vi "Logger Write.vi"(6 "Extra":string, 8 "error in (no error)":errorcluster, 9 "Command":string, 10 "State":string, 11 "Logger in":refnum<class "Logger.lvclass">) -> (0 "error out":errorcluster)   [LabVIEW 2019, in "TS Framework.lvlib" / "Logger.lvclass"]
uses:
  Logger.lvclass
  Logger.lvclass/Logger.ctl
  <vilib>/Utility/error.llb/DialogType.ctl
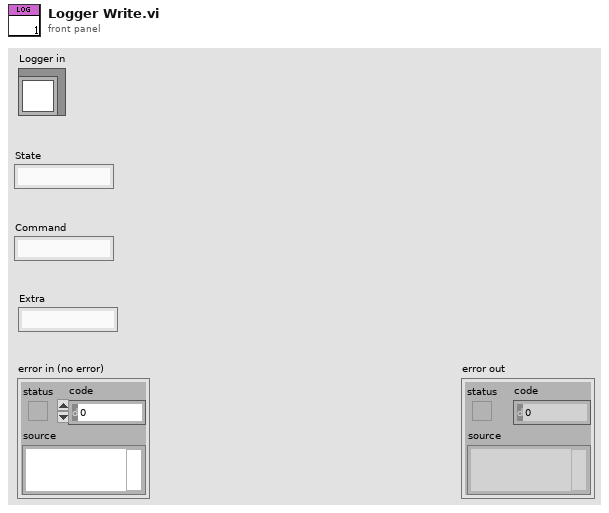
[diagram p1: front panel]
types:
  T1 = typedef "DialogType.ctl" = u16
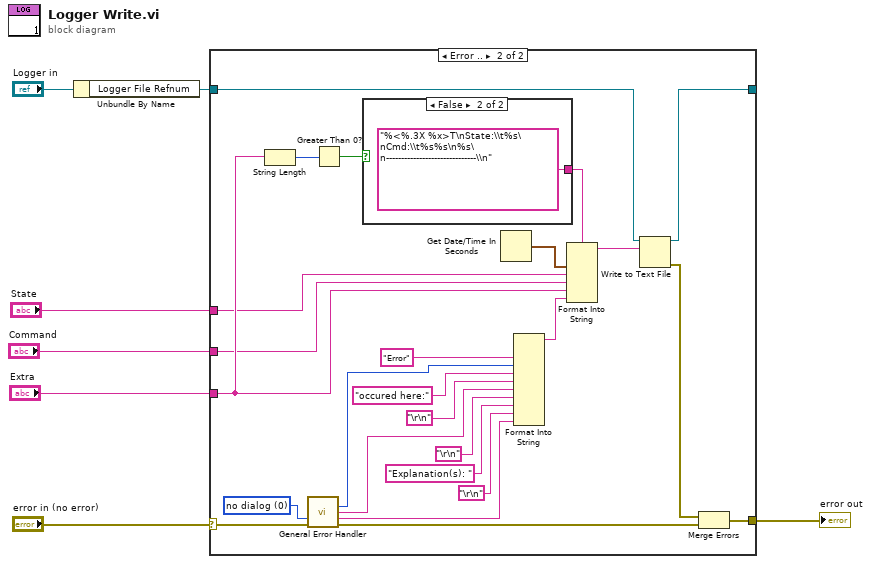
[diagram p0: block diagram]
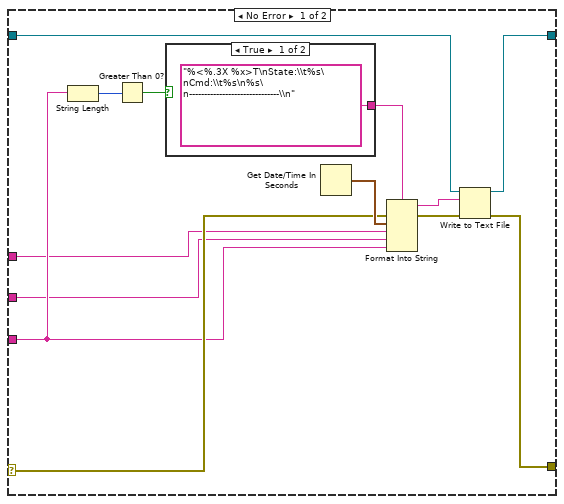
[diagram p2: hidden frame]
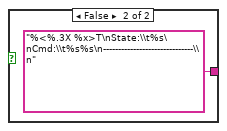
[diagram p3: hidden frame]
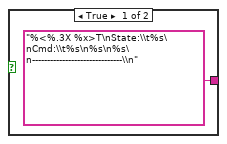
[diagram p4: hidden frame]
diagram:
  n1 = Unbundle By Name("Logger in") -> ("Logger File Refnum"=w5:refnum<file>)
  n2 = case shown="Error .." "error in (no error)" {
    selector: "error in (no error)" -> [w13 w36]
    tunnel: w5 -> [w17 w38]
    tunnel: [w16 w37] -> _
    tunnel: [w15 w33] -> w2
    tunnel: "Extra" -> [w10 w28]
    tunnel: "State" -> [w9 w25]
    tunnel: "Command" -> [w8 w26]
    frame No Error {
      n3 = String Length(string=w10) -> (length=w11:i32)
      n4 = Greater Than 0?(x=w11) -> (x > 0?=w12:bool)
      n5 = case shown="True" w12 {
        tunnel: ["%<%.3X %x>T\nState:\\t%s\nCmd:\\t%s\n%s\n------------------------------\\n" ("format string") "%<%.3X %x>T\nState:\\t%s\nCmd:\\t%s%s\n------------------------------\\n" ("format string")] -> w18
        frame True {
        }
        frame False {
        }
      }
      n6 = Get Date/Time In Seconds() -> (seconds since 1Jan1904=w19:timestamp)
      n7 = Format Into String(format string=w18, error in=w13, w19, w9, w8, w10) -> (resulting string=w20:string, error out=w14:errorcluster)  [unwired: 1 in]
      n8 = Write to Text File(file (use dialog)=w17, text=w20, error in=w14) -> (refnum out=w16:refnum<file>, error out=w15:errorcluster)  [unwired: 1 in, 1 out]
    }
    frame Error {
      w24 = T1 0 items=["no dialog", "OK message", "continue or stop message", "OK message + warnings", "continue/stop + warnings"] ("type of dialog (OK msg:1)")
      n9 = String Length(string=w28) -> (length=w29:i32)
      n10 = call <vilib>:"General Error Handler.vi"("type of dialog (OK msg:1)"=w24, "error in (no error)"=w36) -> ("code out"=w34:i32, "source out"=w23:string, "message"=w45:string, "error out"=w31:errorcluster)  [unwired: 9 in, 1 out]
      n11 = Greater Than 0?(x=w29) -> (x > 0?=w30:bool)
      n12 = case shown="False" w30 {
        tunnel: ["%<%.3X %x>T\nState:\\t%s\nCmd:\\t%s\n%s\n%s\n------------------------------\\n" ("format string") "%<%.3X %x>T\nState:\\t%s\nCmd:\\t%s%s\n%s\n------------------------------\\n" ("format string")] -> w27
        frame True {
        }
        frame False {
        }
      }
      n13 = Get Date/Time In Seconds() -> (seconds since 1Jan1904=w47:timestamp)
      n14 = Format Into String("Error", w34, "occured here:" ("input 3"), "\r\n", w23, "\r\n", "Explanation(s): ", "\r\n", w45) -> (resulting string=w35:string)  [unwired: 3 in, 1 out]
      n15 = Format Into String(format string=w27, w47, w25, w26, w28, w35) -> (resulting string=w46:string)  [unwired: 2 in, 1 out]
      n16 = Write to Text File(file (use dialog)=w38, text=w46) -> (refnum out=w37:refnum<file>, error out=w32:errorcluster)  [unwired: 2 in, 1 out]
      n17 = Merge Errors(w32, w31) -> (w33:errorcluster)
    }
  }
  "error out" <- w2
